vi "Update Points to Acquire.vi"(10 "Points to Acquire":u16, 11 "Trig Offset":u8) -> (2 "Updated Points to Acquire":u16, 3 "Is Trig Offset =0?":bool)   [LabVIEW 2011]
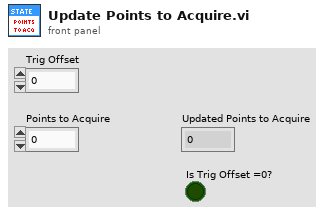
[diagram p1: front panel]
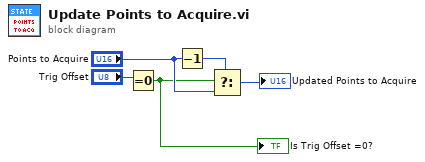
[diagram p0: block diagram]
diagram:
  n1 = Equal To 0?(x="Trig Offset") -> (x = 0?=w1:bool)
  "Is Trig Offset =0?" <- w1
  n2 = Decrement(x="Points to Acquire") -> (x-1=w5:u16)
  n3 = Select(t=w5, s=w1, f="Points to Acquire") -> (s? t:f=→"Updated Points to Acquire":u16)
